vi "Multiply to color convert.vi"() -> ()   [LabVIEW 2018]
uses:
  Multiply.ctl
  Resistor Band Colors.lvlib
panel:
  in  "Multiply":T1
  out "Color":u32
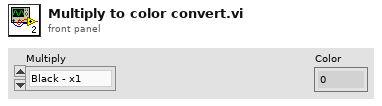
[diagram p1: front panel]
types:
  T1 = typedef "Multiply.ctl" = enum16{"Black - x1", "Brown - x10", "Red - x100", "Orange - x1.000", "Yellow - x10.000", "Green - x100.000", "Blue - x1.000.000", "Violet -  x 10.000.000", "Grey - x100.000.000", "White - x1.000.000.000", "Silver x - 0,01", "Gold x - 0,1"}
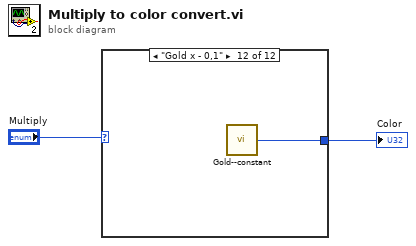
[diagram p0: block diagram]
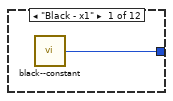
[diagram p2: hidden frame]
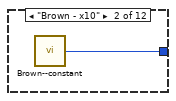
[diagram p3: hidden frame]
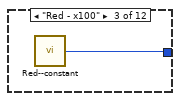
[diagram p4: hidden frame]
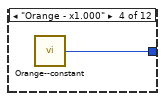
[diagram p5: hidden frame]
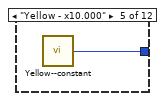
[diagram p6: hidden frame]
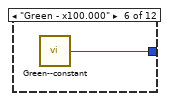
[diagram p7: hidden frame]
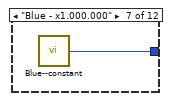
[diagram p8: hidden frame]
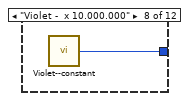
[diagram p9: hidden frame]
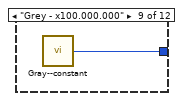
[diagram p10: hidden frame]
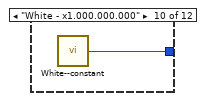
[diagram p11: hidden frame]
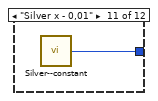
[diagram p12: hidden frame]
diagram:
  n1 = case shown="\"Gold x - 0,1\"" "Multiply" {
    tunnel: [w3 w4 w5 w6 w7 w8 w9 w10 w11 w12 w13 w14] -> w2
    frame "Black - x1" {
      n2 = call "black--constant.vi"() -> ("Color"=w3:u32)  [unwired: 5 in]
    }
    frame "Brown - x10" {
      n3 = call "Brown--constant.vi"() -> ("Color"=w4:u32)  [unwired: 5 in]
    }
    frame "Red - x100" {
      n4 = call "Red--constant.vi"() -> ("Color"=w5:u32)  [unwired: 5 in]
    }
    frame "Orange - x1.000" {
      n5 = call "Orange--constant.vi"() -> ("Color"=w6:u32)  [unwired: 5 in]
    }
    frame "Yellow - x10.000" {
      n6 = call "Yellow--constant.vi"() -> ("Color"=w7:u32)  [unwired: 5 in]
    }
    frame "Green - x100.000" {
      n7 = call "Green--constant.vi"() -> ("Color"=w8:u32)  [unwired: 5 in]
    }
    frame "Blue - x1.000.000" {
      n8 = call "Blue--constant.vi"() -> ("Color"=w9:u32)  [unwired: 5 in]
    }
    frame "Violet -  x 10.000.000" {
      n9 = call "Violet--constant.vi"() -> ("Color"=w10:u32)  [unwired: 5 in]
    }
    frame "Grey - x100.000.000" {
      n10 = call "Gray--constant.vi"() -> ("Color"=w11:u32)  [unwired: 5 in]
    }
    frame "White - x1.000.000.000" {
      n11 = call "White--constant.vi"() -> ("Color"=w12:u32)  [unwired: 5 in]
    }
    frame "Silver x - 0,01" {
      n12 = call "Silver--constant.vi"() -> ("Color"=w13:u32)  [unwired: 5 in]
    }
    frame "Gold x - 0,1" {
      n13 = call "Gold--constant.vi"() -> ("Color"=w14:u32)  [unwired: 5 in]
    }
  }
  "Color" <- w2
